vi "IT6322_Config.vi"(6 "等待时间(毫秒)":u32=100, 7 "设置值":dbl=15.0, 8 "error in":errorcluster caption="错误输入（无错误）", 9 "通道选择":enum16{"第一通道", "第二通道", "第三通道"}(ring), 10 "电压电流":enum16{"VOLTage", "CURR"}(ring), 11 "MyIndex":u8) -> (0 "error out":errorcluster, 2 "返回值":string, 3 "状态":bool)   [LabVIEW 2015, in "IT6322.lvlib"]
uses:
  IT6322.lvlib
  <vilib>/Instr/_visa.llb/VISA Configure Serial Port (Instr).vi
panel:
  out "VISA":refnum<visa-resource-name>
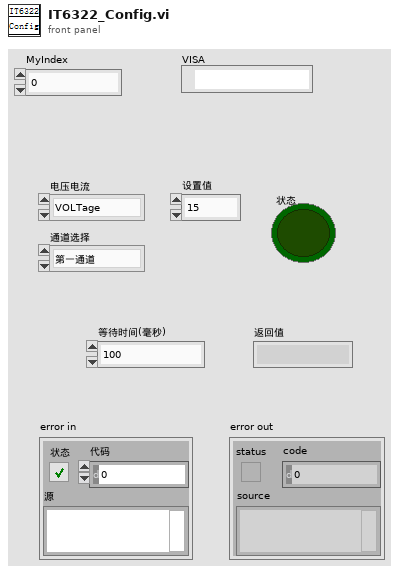
[diagram p1: front panel]
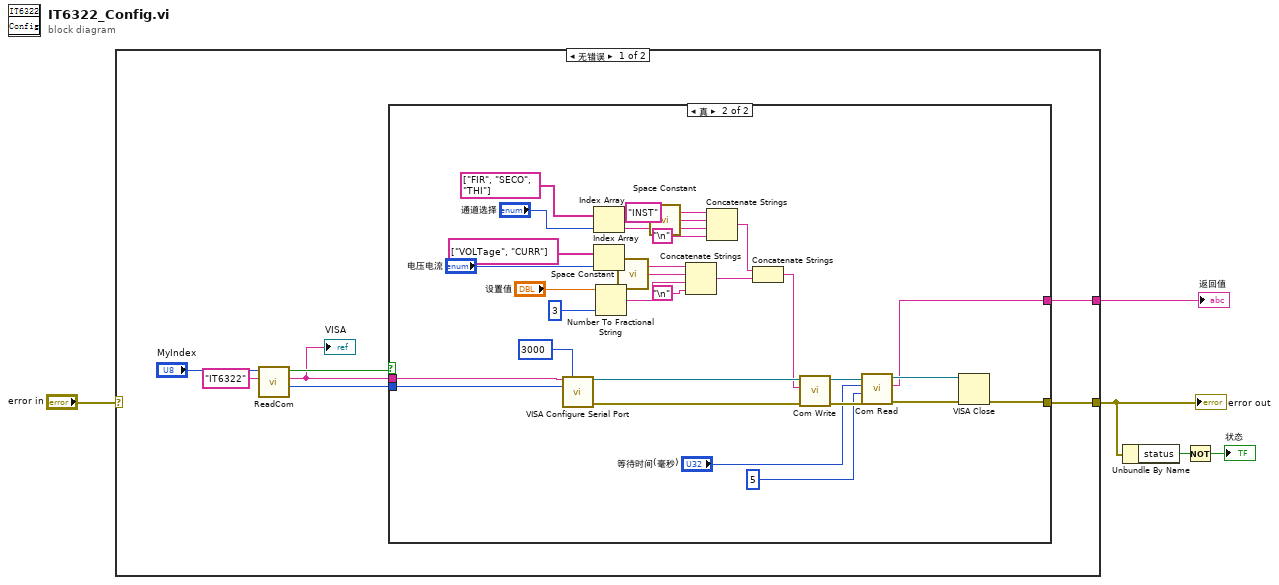
[diagram p0: block diagram]
diagram:
  n1 = case shown="无错误" "error in" {
    selector: "error in" -> [_ w43]
    tunnel: [w12 w43] -> w2
    tunnel: [w6 _] -> w3
    frame No Error {
      n2 = call "ReadCom.vi"("仪器名称"="IT6322", "MyIndex"="MyIndex") -> ("Baudrate"=w7:i32, "COM"=w8:string, "OK?"=w9:bool)  [unwired: 7 in]
      "VISA" <- w8
      n3 = case shown="真" w9 {
        tunnel: [_ w42] -> w12
        tunnel: w8 -> [_ w41]
        tunnel: w7 -> [_ w40]
        tunnel: [_ w32] -> w6
        frame False {
        }
        frame True {
          n4 = call-poly "VISA Configure Serial Port"("VISA resource name"=w41, "timeout (10sec)"=u32 3000, "baud rate (9600)"=w40) -> ("VISA resource name out"=w38:refnum<visa-resource-name>, "error out"=w37:errorcluster)  [unwired: 11 in]
          n5 = Index Array(array=string[] ["FIR", "SECO", "THI"], index="通道选择") -> (element=w25:string)
          n6 = Index Array(array=string[] ["VOLTage", "CURR"], index="电压电流") -> (element=w28:string)
          n7 = Number To Fractional String(number="设置值", precision (6)=i16 3 ("精度(6)")) -> (F-format string=w16:string)  [unwired: 2 in]
          n8 = call <vilib>:"Space Constant.vi"() -> ("String"=w15:string)
          n9 = call <vilib>:"Space Constant.vi"() -> ("String"=w20:string)
          n10 = Concatenate Strings(w28, w15, w16, "\n") -> (w23:string)
          n11 = Concatenate Strings("INST", w20, w25, "\n") -> (w22:string)
          n12 = Concatenate Strings(w22, w23) -> (w13:string)
          n13 = call "Com Write.vi"("错误输入（无错误）"=w37, "Wbuff"=w13, "VISA In"=w38) -> ("错误输出"=w35:errorcluster, "VISA Out"=w36:refnum<visa-resource-name>)  [unwired: 7 in]
          n14 = call "Com Read.vi"("错误输入（无错误）"=w35, "num"=u32 5, "超时"="等待时间(毫秒)", "VISA In"=w36) -> ("错误输出"=w34:errorcluster, "buff"=w32:string, "VISA Out"=w33:refnum<visa-resource-name>)  [unwired: 5 in]
          n15 = VISA Close(VISA resource name=w33, error in (no error)=w34) -> (error out=w42:errorcluster)
        }
      }
    }
    frame Error {
    }
  }
  "error out" <- w2
  "返回值" <- w3
  n16 = Unbundle By Name(w2) -> ("status"=w1:bool)
  n17 = Not(x=w1) -> (.not. x?=→"状态":bool)
